vi "DAQmx_Pulse_Train.vi"(0 "Counter(s)":tag="Dev1/ctr1", 1 "Start?":bool, 3 "Frequency":dbl=1.0 caption="Frequency (Hz)" format="%0.2f", 5 "Duty Cycle":dbl=0.5 min=0.0 max=1.0 format="%0.2f") -> ()   [LabVIEW 2010]
doc: "I. Description:\nThis example demonstrates how to generate a continuous digital pulse train from a Counter Output Channel. The Frequency, Duty Cycle, and Idle State are all configurable. \n\nThis example shows how to configure the pulse in terms of Frequency/Duty Cycle, but can easily be modified to generate a pulse in terms of Time or Ticks.\n\nII. Instructions for Running:\n1. Select the Physical Channel which corresponds to the counter you want to output your signal to on the DAQ device.\n2. Enter the Frequency and Duty Cycle to define the pulse parameters. You can also change the Idle State to determine the beginning and end states of the output. If the Idle State is High, the generation will use inverted logic. Additionally, you can set the Initial Delay (in seconds) which will delay the beginning of the pulse train from the start call; this is currently wired to 0.0 on the diagram. \nNote: Use the Measure Period example to verify you are outputting the pulse train on the DAQ device.\n\nIII. Block Diagram Steps:\n1. Create an empty task\n2. Create a Counter Output channel to produce a Pulse in terms of Frequency. If the Idle State of the pulse is set to low, the state of the line will begin low and remain low after the generation is stopped.\n3. Use the DAQmx Base Timing VI (Implicit) to configure the duration of the pulse generation.\n4. Call the Start VI to arm the counter and begin the pulse train generation.\n5. Loop continuously until the user presses the Stop button. Check for errors every 100 ms using the Is Task Done? VI\n6. Stop the task\n7. Clear the Task.\n\nIV. I/O Connections Overview:\nThe counter will output the pulse train on the output terminal of the counter specified in the Physical Channel I/O control. \n\nIn this example the output will be sent to the default output terminal on ctr0.\n\nFor more information on the default counter input and output terminals for your device, open the NI-DAQmx Help, and refer to Counter Signal Connections found under the Device Considerations book in the table of contents."
uses:
  <vilib>/_DAQmxBase/Internals/DAQmxBase Create Channel (CO-Pulse Generation-Frequency).vi
  <vilib>/_DAQmxBase/Internals/DAQmxBase Timing (Implicit).vi
panel:
  # "For instructions, select Help>>Show Context Help"
  # "Channel Parameters"
  # "Wire to Chip in the connection box\nneed connecting to OUT 1"
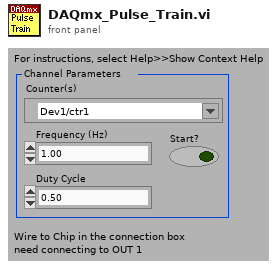
[diagram p1: front panel]
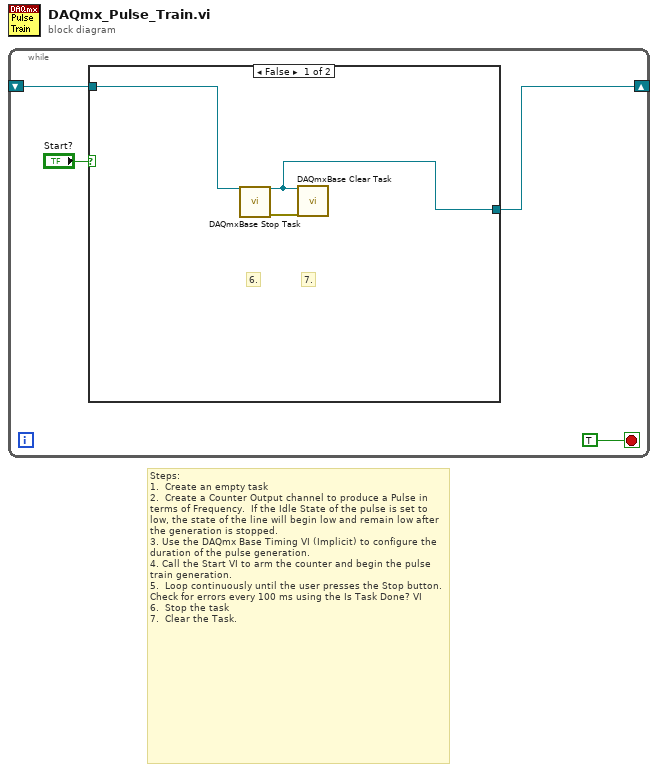
[diagram p0: block diagram]
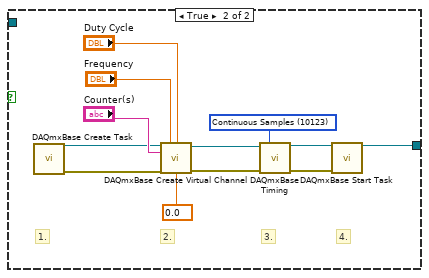
[diagram p2: hidden frame]
diagram:
  # "Steps: \n1.  Create an empty task\n2.  Create a Counter Output channel to produce a Pulse in terms of Frequency.  If the Idle State of the pulse is set to low, the state of the line will begin low and remain low after the generation is stopped.\n3. Use the DAQmx Base Timing VI (Implicit) to configure the duration of the pulse generation.\n4. Call the Start VI to arm the counter and begin the pulse train generation.\n5.  Loop continuously until the user presses the Stop button. Check for errors every 100 ms using the Is Task Done? VI\n6.  Stop the task\n7.  Clear the Task."
  n1 = while {
    shift-right: [w4] -> _
    shift-left: _ -> [w2]
    stop <- TRUE stop-if-true
    n2 = case shown="False" "Start?" {
      tunnel: [w5 w8] -> w4
      tunnel: w2 -> [w6 _]
      frame False {
        # "7."
        # "6."
        n3 = call <vilib>:"DAQmxBase Stop Task.vi"("task/channels in"=w6) -> ("task out"=w5:refnum<k21>, "error out"=w7:errorcluster)  [unwired: 13 in]
        n4 = call <vilib>:"DAQmxBase Clear Task.vi"("task in"=w5, "error in"=w7) -> ()  [unwired: 13 in, 1 out]
      }
      frame True {
        w15 = 10123 items=["Finite Samples"=10178, "Continuous Samples"=10123] ("sample mode")
        # "4."
        # "3."
        # "2."
        # "1."
        n5 = call <vilib>:"DAQmxBase Create Task.vi"() -> ("task out"=w9:refnum<k21>, "error out"=w10:errorcluster)  [unwired: 14 in]
        n6 = call-poly <vilib>:"DAQmxBase Create Virtual Channel.vi"("task in"=w9, "frequency"="Frequency", "duty cycle"="Duty Cycle", "counter"="Counter(s)", "error in"=w10, "initial delay"=0.0) -> ("task out"=w18:refnum<k21>, "error out"=w19:errorcluster)  [unwired: 8 in]
        n7 = call-poly <vilib>:"DAQmxBase Timing.vi"("task/channels in"=w18, "sample mode"=w15, "error in"=w19) -> ("task out"=w16:refnum<k21>, "error out"=w17:errorcluster)  [unwired: 11 in]
        n8 = call <vilib>:"DAQmxBase Start Task.vi"("task/channels in"=w16, "error in"=w17) -> ("task out"=w8:refnum<k21>)  [unwired: 12 in, 1 out]
      }
    }
  }
